vi "stamm.vi"(10 "Height":sgl, 11 "Radius":sgl) -> (0 "Fehler (Ausgang)":errorcluster, 3 "SceneObject (Ausgang)":refnum<vi>)   [LabVIEW 2014]
uses:
  <vilib>/picture/3D Picture Control/Object/Create Object (drawable).vi
  <vilib>/picture/3D Picture Control/NI_3D Picture Control.lvlib
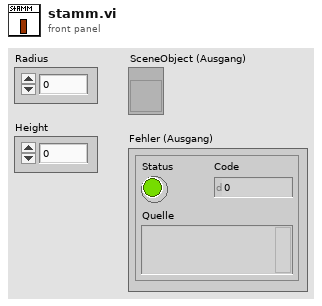
[diagram p1: front panel]
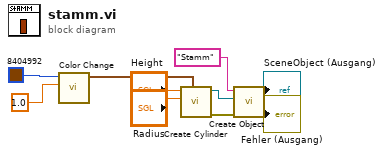
[diagram p0: block diagram]
diagram:
  n1 = call <vilib>:"Color Change.vi"("Alpha"=1.0, "Color"=u32 8404992) -> ("RGBA"=w10:cluster{"R":sgl, "G":sgl, "B":sgl, "A":sgl})  [unwired: 9 in]
  n2 = call <vilib>:"Create Cylinder.vi"("Color"=w10, "Radius"="Radius", "Height"="Height") -> ("error out"=w5:errorcluster, "New Cylinder Refnum"=w3:refnum<vi>)  [unwired: 7 in]
  n3 = call-poly <vilib>:"Create Object.vi"("error in (no error)"=w5, "Geometry"=w3, "Name"="Stamm") -> ("error out"=→"Fehler (Ausgang)":errorcluster, "Scene:New Object"=→"SceneObject (Ausgang)":refnum<vi>)  [unwired: 7 in]
